vi "Distance Test.vi"(9 "Camera view angle":dbl format="%#_13g", 10 "Rectangle":T1, 11 "Y Image Resolution":i32) -> (2 "Distance (cm)":dbl)   [LabVIEW 2013]
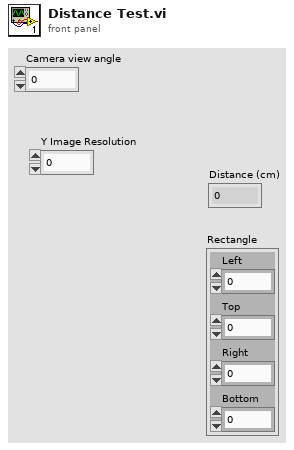
[diagram p1: front panel]
types:
  T1 = cluster{"Left":dbl, "Top":dbl, "Right":dbl, "Bottom":dbl}
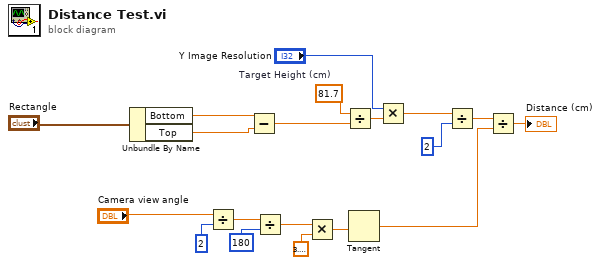
[diagram p0: block diagram]
diagram:
  w13 = 81.7  # Target Height (cm)
  n1 = Unbundle By Name("Rectangle") -> ("Bottom"=w6:dbl, "Top"=w5:dbl)
  n2 = Divide(x="Camera view angle", y=2) -> (x/y=w10:dbl)
  n3 = Subtract(x=w6, y=w5) -> (x-y=w4:dbl)
  n4 = Divide(x=w10, y=180) -> (x/y=w11:dbl)
  n5 = Multiply(x=w11, y=3.141592653589793) -> (x*y=w9:dbl)
  n6 = Divide(x=w13, y=w4) -> (x/y=w14:dbl)
  n7 = Tangent(1:w9) -> (0:w18:dbl)
  n8 = Multiply(x="Y Image Resolution", y=w14) -> (x*y=w3:dbl)
  n9 = Divide(x=w3, y=2) -> (x/y=w17:dbl)
  n10 = Divide(x=w17, y=w18) -> (x/y=→"Distance (cm)":dbl)
